vi "Hierarchical Clustering.vi"() -> ()   [LabVIEW 2020]
doc: "Example builds a swiss roll dataset and runs hierarchical clustering on their position."
uses:
  Model/Unsupervised/Cluster/AgglomerativeClustering/controls/agglomerative_clustering_params.ctl
  <vilib>/Math Plots/3D Math Plots/3D Scatter/3D Scatter XCtrl/3D Scatter.xctl
  <vilib>/Math Plots/3D Math Plots/3D Plot/3D Plot Datatype/3D Plot Datatype.lvclass
  PLAIYDISPLAY/Display/_Controls/Style.ctl
  Model/Unsupervised/Cluster/AgglomerativeClustering/AgglomerativeClustering.lvclass
  C:/Users/cipop/TDF Dropbox/2_Technologies de France/1 - Services et Etudes/PLAIY/2 - DEV/PLAIYLAB/code/Model/Model.lvclass
  Model/Unsupervised/Cluster/AgglomerativeClustering/AgglomerativeClustering.vi
panel:
  out "error out":errorcluster
  out "3D Scatter":refnum<class "3D Plot Datatype.lvclass">[](xcontrol)
  out "labels_":dbl[](array[numeric])
  in  "R/W params":T1={"n_clusters"={"n_clusters_type"="int", "n_clusters_int"=6.0}, "affinity"={"affinity_type"="euclidean", "affinity_function"="metric_function"}, "memory"="", "connectivity"={"connectivity_type"="None", "connectivity_list"=[]}, "compute_full_tree"={"compute_full_tree_type"="auto", "compute_full_tree_bool"=FALSE}, "linkage"="ward", "distance_threshold"={"distance_threshold_type"="None", "distance_threshold_float"=0.0}, "compute_distances"=FALSE}
  out "Array":dbl[](array[numeric])
  out "X":dbl[][](array[numeric])
  in  "error in (no error)":errorcluster caption="entrée d'erreur (pas d'erreur)"
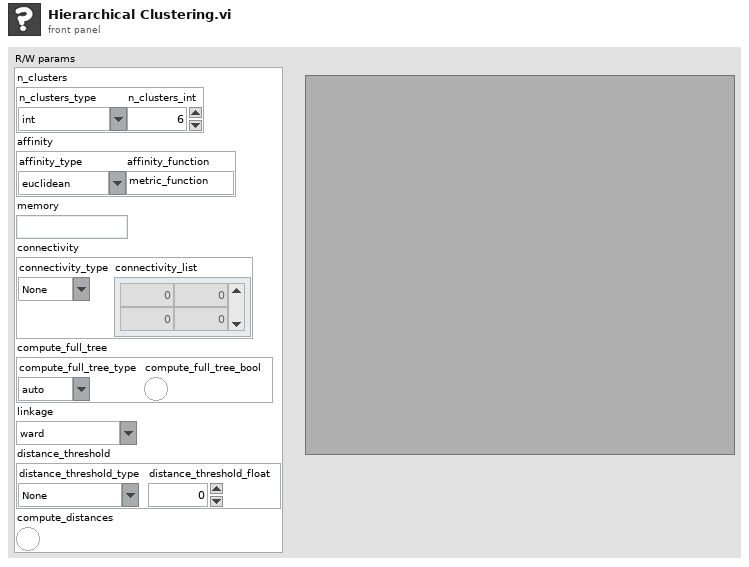
[diagram p1: front panel]
types:
  T1 = typedef "agglomerative_clustering_params.ctl" = cluster{"n_clusters":cluster{"n_clusters_type":string, "n_clusters_int":dbl}, "affinity":cluster{"affinity_type":string, "affinity_function":string}, "memory":string, "connectivity":cluster{"connectivity_type":string, "connectivity_list":dbl[][]}, "compute_full_tree":cluster{"compute_full_tree_type":string, "compute_full_tree_bool":bool}, "linkage":string, "distance_threshold":cluster{"distance_threshold_type":string, "distance_threshold_float":dbl}, "compute_distances":bool}
  T2 = typedef "Style.ctl" = enum16{"Empty circle", "Full circle", "Empty square", "Full square", "Cross"}
  T3 = cluster{"Parameter":cluster{"3D Plot":refnum<class "3D Plot Datatype.lvclass">[], "3D Scatter":refnum<vi>, "Data":cluster{"X":dbl[][], "Predict":dbl[][]}, "Display":cluster{"Choice":enum16{"All", "Train", "Test"}, "Indexe":cluster{"X":i32, "Y":i32, "Z":i32}}, "Point Property":cluster{"Style":T2, "Label Color":u32[]}}}
  T4 = cluster{"n_samples":u32, "noise":dbl, "random_state":i32, "Returns":string}
  T5 = cluster{" 4DArray":cluster{"1":string[][], "2":string[][]}[], " 3DArray":cluster{"Tableau":string[][]}[], "Sparse Matrix 2DArray":string[][], " 2DArray":string[][], " 1DArray":string[]}
  T6 = typedef "agglomerative_clustering_attributes.ctl" = cluster{"n_clusters_":dbl, "labels_":dbl[], "n_leaves_":dbl, "n_connected_components_":dbl, "children_":dbl[][], "distances_":dbl[]}
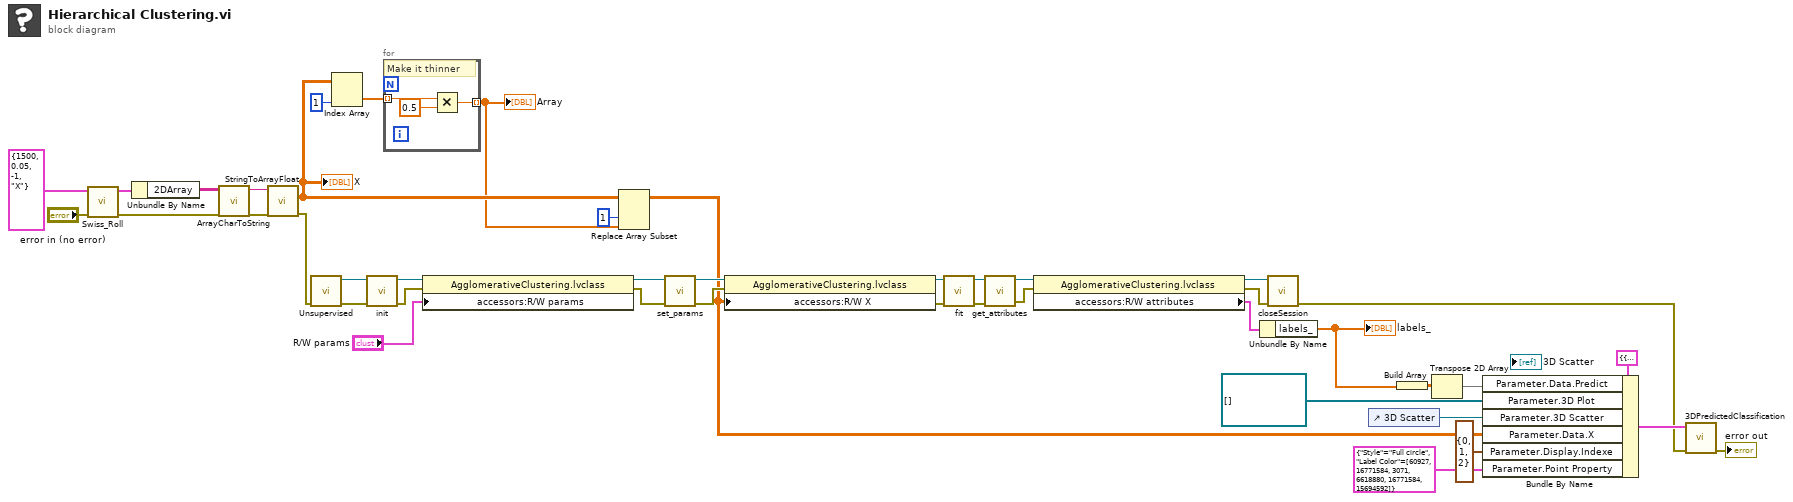
[diagram p0: block diagram]
diagram:
  n1 = call "Swiss_Roll.vi"("error in (no error)"="error in (no error)", "make_swiss_roll"=T4 {"n_samples"=1500, "noise"=0.05, "random_state"=-1, "Returns"="X"}) -> ("error out"=w37:errorcluster, "Data"=w40:T5)  [unwired: 8 in]
  n2 = Unbundle By Name(w40) -> ("2DArray"=w38:string[][])
  n3 = call "ArrayCharToString.vi"("TAB"=w38) -> ("Instruction"=w39:string)  [unwired: 10 in]
  n4 = call "StringToArrayFloat.vi"("entrée d'erreur (pas d'erreur)"=w37, "Return value"=w39) -> ("error IO"=w20:errorcluster, "2DArray"=w5:dbl[][])  [unwired: 7 in, 1 out]
  "X" <- w5
  n5 = call-poly "Unsupervised.vi"("error in"=w20) -> ("error out"=w21:errorcluster, "out"=w22:refnum<class "AgglomerativeClustering.lvclass">)  [unwired: 9 in]
  n6 = Index Array(array=w5, index (col)=1 ("disabled index (col)")) -> (element=w35:dbl[])  [unwired: 1 in]
  n7 = call-dynamic "init.vi"("error in (no error)"=w21, "Model en entrée"=w22) -> ("error out"=w28:errorcluster, "Model en sortie"=w32:refnum<class "AgglomerativeClustering.lvclass">)  [unwired: 8 in]
  n8 = for {
    tunnel: w35 -> [w45] mode=indexing
    tunnel: [w43] -> w3 mode=indexing
    # "Make it thinner"
    n9 = Multiply(x=w45, y=0.5) -> (x*y=w43:dbl)
  }
  "Array" <- w3
  n10 = property class="AgglomerativeClustering.lvclass"(reference=w32, error in=w28, "accessors:R/W params"="R/W params") -> (reference out=w31:refnum<class "AgglomerativeClustering.lvclass">, error out=w19:errorcluster)
  n11 = Replace Array Subset(array=w5, new element=w3, index (col)=1 ("disabled index (col)")) -> (w4:dbl[][])  [unwired: 1 in]
  n12 = call-dynamic "set_params.vi"("error in (no error)"=w19, "AgglomerativeClustering.lvclass 2"=w31) -> ("error out"=w29:errorcluster, "AgglomerativeClustering.lvclass"=w30:refnum<class "AgglomerativeClustering.lvclass">)  [unwired: 8 in]
  n13 = property class="AgglomerativeClustering.lvclass"(reference=w30, error in=w29, "accessors:R/W X"=w4) -> (reference out=w34:refnum<class "AgglomerativeClustering.lvclass">, error out=w33:errorcluster)
  n14 = call-dynamic "fit.vi"("error in (no error)"=w33, "AgglomerativeClustering.lvclass 2"=w34) -> ("error out"=w25:errorcluster, "AgglomerativeClustering.lvclass"=w26:refnum<class "AgglomerativeClustering.lvclass">)  [unwired: 8 in]
  n15 = call-dynamic "get_attributes.vi"("error in (no error)"=w25, "AgglomerativeClustering.lvclass 2"=w26) -> ("error out"=w6:errorcluster, "AgglomerativeClustering.lvclass"=w7:refnum<class "AgglomerativeClustering.lvclass">)  [unwired: 8 in]
  n16 = property class="AgglomerativeClustering.lvclass"(reference=w7, error in=w6) -> (reference out=w27:refnum<class "AgglomerativeClustering.lvclass">, error out=w18:errorcluster, "accessors:R/W attributes"=w24:T6)
  n17 = Unbundle By Name(w24) -> ("labels_"=w9:dbl[])
  "labels_" <- w9
  n18 = call-dynamic "closeSession.vi"("error in"=w18, "Python en entrée"=w27) -> ("error out"=w8:errorcluster)  [unwired: 8 in, 1 out]
  n19 = control-ref of="3D Scatter"() -> (w10:refnum<vi>)
  n20 = Build Array(w9) -> (w12:dbl[][])
  n21 = Transpose 2D Array(2D array=w12) -> (transposed array=w11:dbl[][])
  n22 = Bundle By Name(cluster=T3 {"Parameter"={"3D Plot"=[], "3D Scatter"=refnum, "Data"={"X"=[], "Predict"=[]}, "Display"={"Choice"=enum."All", "Indexe"={"X"=0, "Y"=1, "Z"=2}}, "Point Property"={"Style"=enum."Full circle", "Label Color"=[8978528, 4367871, 1985280]}}} ("Parameters"), "Parameter.Data.Predict"=w11, "Parameter.3D Plot"=refnum<class "3D Plot Datatype.lvclass">[] [] ("3D Scatter"), "Parameter.3D Scatter"=w10, "Parameter.Data.X"=w4, "Parameter.Display.Indexe"=cluster{"X":i32, "Y":i32, "Z":i32} {"X"=0, "Y"=1, "Z"=2}, "Parameter.Point Property"=cluster{"Style":T2, "Label Color":u32[]} {"Style"=enum."Full circle", "Label Color"=[60927, 16771584, 3071, 6618880, 16771584, 15694592]} ("Point Property")) -> (w13:T3)
  n23 = call "3DPredictedClassification.vi"("error in"=w8, "Parameters"=w13) -> ("error out"=→"error out":errorcluster)  [unwired: 8 in, 1 out]
